vi "Get ActiveCell Pos.vi"(8 "error in (no error)":errorcluster caption="错误输入（无错误）", 11 "Table Ref In":refnum<vi>) -> (0 "error out":errorcluster caption="错误输出", 2 "ActiveCell Pos":T1 caption="活动单元格:位置", 3 "Table Ref Out":refnum<vi>)   [LabVIEW 2013, in "Table Tool.lvlib"]
uses:
  Table Tool.lvlib
  <vilib>/Utility/miscctls.llb/LVPositionTypeDef.ctl
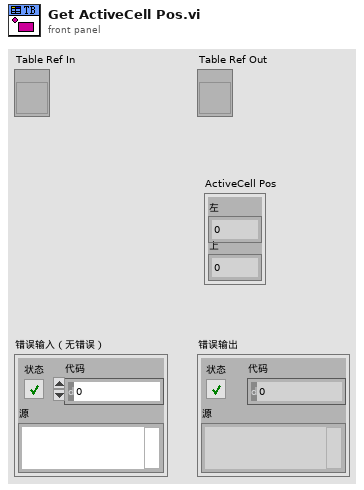
[diagram p1: front panel]
types:
  T1 = typedef "LVPositionTypeDef.ctl" = cluster{"Left":i32, "Top":i32}
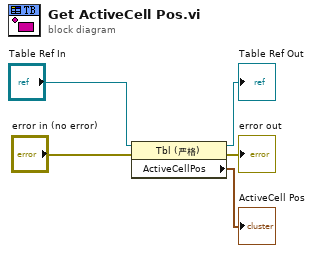
[diagram p0: block diagram]
diagram:
  n1 = property class="Tbl (严格)"(reference="Table Ref In", error in="error in (no error)") -> (reference out=→"Table Ref Out":refnum<vi>, error out=→"error out":errorcluster, "ActiveCellPos"=→"ActiveCell Pos":T1)
